vi "LVtoISO8601.vi"(1 "Labview Timestamp":timestamp) -> (0 "ISO8601 Timestamp":string)   [LabVIEW 2013, in "SetListPrefs.lvclass"]
uses:
  SetListPrefs.lvclass
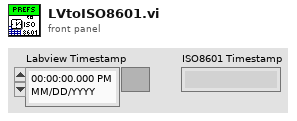
[diagram p1: front panel]
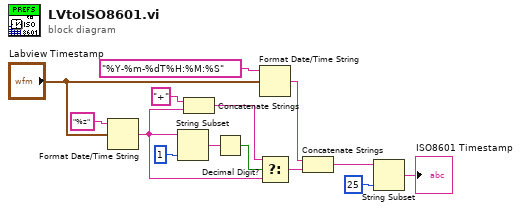
[diagram p0: block diagram]
diagram:
  n1 = Format Date/Time String(time format string (%c)="%z", seconds (now)="Labview Timestamp") -> (date/time string=w11:string)  [unwired: 1 in]
  n2 = String Subset(string=w11, length (rest)=1 ("length (rest)")) -> (substring=w7:string)  [unwired: 1 in]
  n3 = Concatenate Strings("+" ("string"), w11) -> (w10:string)
  n4 = Decimal Digit?(1:w7) -> (0:w9:bool)
  n5 = Format Date/Time String(time format string (%c)="%Y-%m-%dT%H:%M:%S", seconds (now)="Labview Timestamp") -> (date/time string=w12:string)  [unwired: 1 in]
  n6 = Select(t=w10, s=w9, f=w11) -> (s? t:f=w13:string)
  n7 = Concatenate Strings(w12, w13) -> (w14:string)
  n8 = String Subset(string=w14, length (rest)=25 ("length (rest)")) -> (substring=→"ISO8601 Timestamp":string)  [unwired: 1 in]
